vi "Set Error Reporting.vi"(8 "error in (no error)":errorcluster, 10 "Error Reporting":T1, 11 "Session in":refnum<class "Session.lvclass">) -> (0 "error out":errorcluster, 3 "Session out":refnum<class "Session.lvclass">)   [LabVIEW 2024, in "CTI.lvlib" / "Session.lvclass"]
doc: "Sets the level of automatic error checking and reporting that occurs during interactions with a device.\n- <b>Full</b>: The device is queried for errors automatically after every interaction and all error checking that has been implemented will be performed.\n-<b>Moderate</b>: Currently no different then <b>Minimal</b> and is a placeholder for future error handling updates.\n-<b>Minimal</b>: The automatic device error querying is not performed and only internal communication handling error checks are typically done."
uses:
  Session.lvclass
  Error Reporting.ctl
  Session.lvclass/Session.ctl
  CTI.lvlib
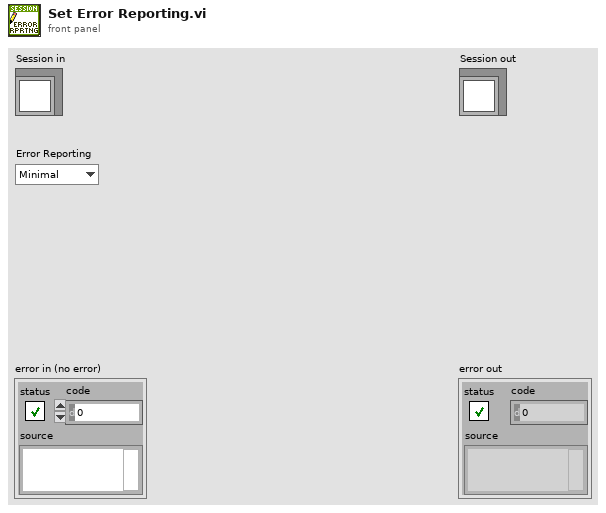
[diagram p1: front panel]
types:
  T1 = typedef "CTI.lvlib/Error Reporting.ctl" = enum16{"Minimal", "Moderate", "Full"}
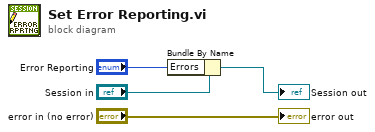
[diagram p0: block diagram]
diagram:
  n1 = Bundle By Name(cluster="Session in", "Errors"="Error Reporting") -> (→"Session out":refnum<class "Session.lvclass">)
  "error out" <- "error in (no error)"
